vi "WorkorderHandler_Create.vi"(7 "object name (unnamed)":string, 8 "error in (no error)":errorcluster) -> (0 "error out":errorcluster, 3 "reference":T1)   [LabVIEW 2011]
uses:
  DataStructures/WorkorderHandler_ObjectReference.ctl
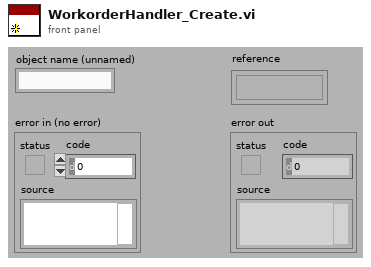
[diagram p1: front panel]
types:
  T1 = typedef "WorkorderHandler_ObjectReference.ctl" = refnum<k1>
  T2 = typedef "WorkorderHandler_ObjectData.ctl" = cluster{"Table":string[][], "Script":string, "Order":string, "No":string, "Time":dbl}
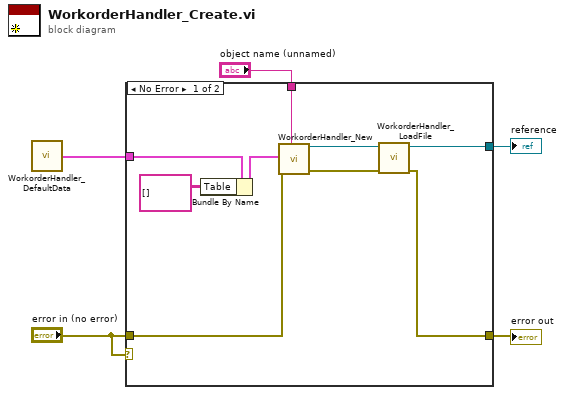
[diagram p0: block diagram]
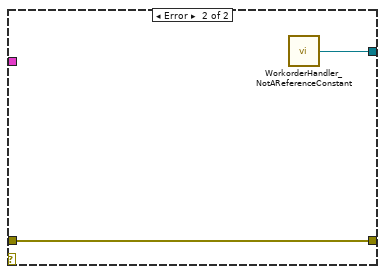
[diagram p2: hidden frame]
diagram:
  n1 = call "WorkorderHandler_DefaultData.vi"() -> ("data"=w3:T2)
  n2 = case shown="No Error" "error in (no error)" {
    tunnel: [w6 w16] -> w5
    tunnel: w3 -> [w13 _]
    tunnel: [w8 w15] -> w4
    tunnel: "error in (no error)" -> [w12 w16]
    tunnel: "object name (unnamed)" -> [w11 _]
    frame No Error {
      n3 = Bundle By Name(cluster=w13, "Table"=string[][] []) -> (w14:T2)
      n4 = call "WorkorderHandler_New.vi"("data"=w14, "error in (no error)"=w12, "object name (unnamed)"=w11) -> ("reference"=w9:T1, "error out"=w7:errorcluster)  [unwired: 1 in, 14 out]
      n5 = call "WorkorderHandler_LoadFile.vi"("error in (no error)"=w7, "reference"=w9) -> ("error out"=w6:errorcluster, "duplicate reference"=w8:T1)  [unwired: 8 out]
    }
    frame Error {
      n6 = call "WorkorderHandler_NotAReferenceConstant.vi"() -> ("reference"=w15:T1)
    }
  }
  "error out" <- w5
  "reference" <- w4
